vi "playback_choose_freq.vi"() -> ()   [LabVIEW 2012]
doc: "This VI will initialize the FPGA VI and read a user-defined number of samples from a DMA FIFO. When the data acquisition is complete this VI will read status information from the FPGA VI.\n\nFollow these instructions to run the VI.\n\n1. Select your RIO device from the dropdown.\n2. Set the sample period, number of samples to acquire per channel, and DMA block read size. \n\nNote: the block read size should be set to balance load on the host processor and the update rate of the user interface. A small block read size will update the user interface more often but will result in a higher load on the host processor."
uses:
  <vilib>/Analysis/3filter.llb/Butterworth Filter (DBL).vi
  <vilib>/Analysis/NI_AALBase.lvlib
panel:
  out "Selected Index":i32
  out "Ratio at Index (%)":dbl
  in  "Threshold":dbl=0.1
  out "Index 0":dbl
  out "Index 1":dbl
  out "Index 2":dbl
  out "Index 3":dbl
  in  "noise min":dbl=0.001
  out "amplitude 0":dbl
  out "amplitude 1":dbl
  out "amplitude 2":dbl
  out "amplitude 3":dbl
  in  "Portion Duration":i32=600
  in  "Altitude":dbl=2.0
  out "x":dbl
  out "y":dbl
  out "z":dbl
  out "yaw":dbl
  out "pitch":dbl
  out "Yaw Chart":dbl(graph)
  in  "Mode":T1(ring)=enum."Use Far Field"
  out "Threshold 0":dbl
  out "Threshold 1":dbl
  out "Threshold 2":dbl
  out "Threshold 3":dbl
  in  "threshold ratio":dbl=3.0
  out "bad signal?":bool
  out "ROS  Error":bool
  in  "Send to ROS":bool
  out "dt1":dbl
  out "dt2":dbl
  out "dt3":dbl
  out "Forward":dbl
  out "Sidemove":dbl
  out "Extracted signal":dbl[][](graph)
  in  "Debug":bool=TRUE
  in  "Select Frequency":dbl=24000.0
  out "frequency 2":dbl
  out "frequency 1":dbl
  out "Chosen Signal":dbl[][](graph)
  in  "Wait?":bool
  in  "Next Signal":bool
  in  "Filename":path=path "D/Recorded/US Test/Robosub day 1/pinger_in_front.tdms"
  out "Original Filtered Ch0":dbl[](graph)
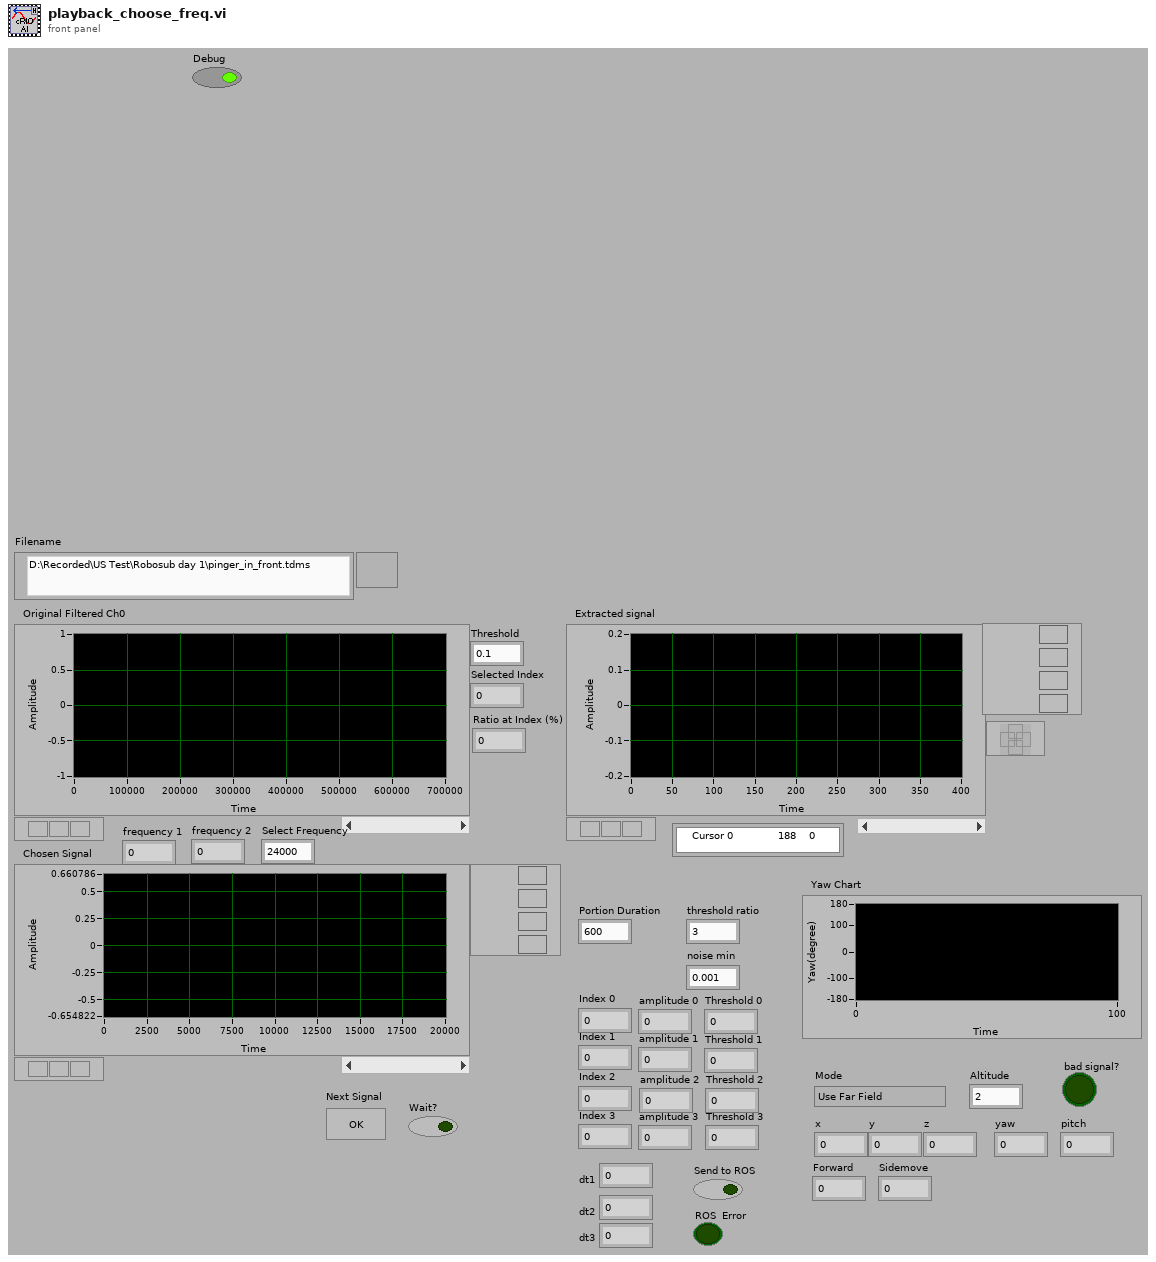
[diagram p1: front panel]
types:
  T1 = enum16{"Use Near Field", "Use Far Field", "Far Field with 3 hydrophones"}
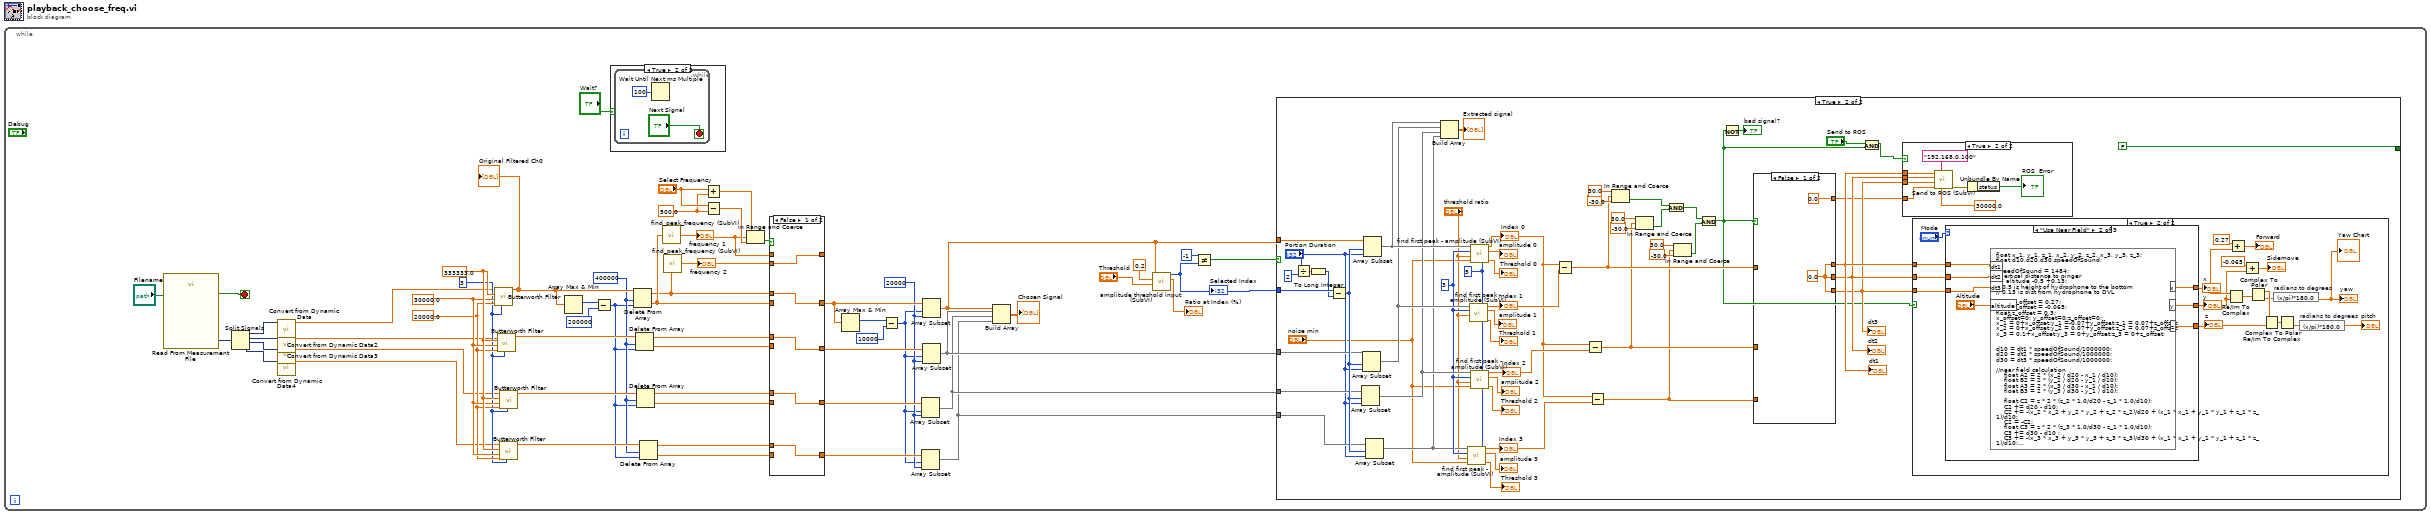
[diagram p0: block diagram]
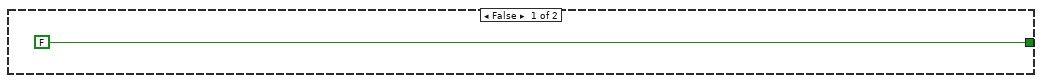
[diagram p2: hidden frame]
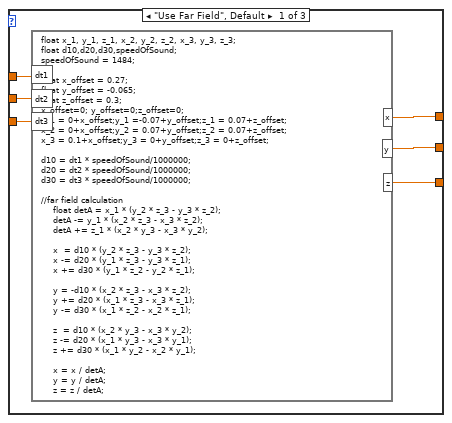
[diagram p4: hidden frame]
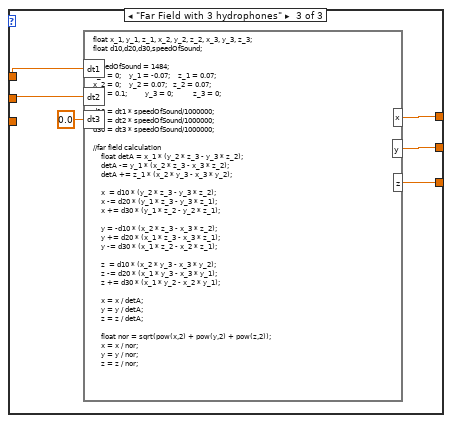
[diagram p5: hidden frame]
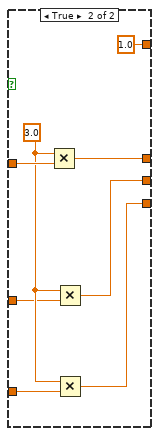
[diagram p7: hidden frame]
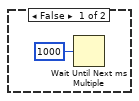
[diagram p8: hidden frame]
diagram:
  n1 = while {
    stop <- w46 stop-if-true
    w17 = 500.0
    w23 = 20000
    w37 = 400000
    w56 = 20000.0
    w57 = 30000.0
    w55 = 3
    w58 = 333333.0
    n2 = call "Read From Measurement File"("Filename"="Filename") -> ("Signals"=w50:dynamicdata, "EOF?"=w46:bool)  [unwired: 5 in, 4 out]
    n3 = Split Signals(w50) -> (w54:dynamicdata, w53:dynamicdata, w52:dynamicdata, w51:dynamicdata)  [unwired: 4 in]
    n4 = call "Convert from Dynamic Data"("Dynamic Data Type"=w54) -> ("Array"=w44:dbl[])  [unwired: 3 in]
    n5 = call "Convert from Dynamic Data2"("Dynamic Data Type"=w53) -> ("Array"=w49:dbl[])  [unwired: 3 in]
    n6 = call "Convert from Dynamic Data3"("Dynamic Data Type"=w52) -> ("Array"=w47:dbl[])  [unwired: 3 in]
    n7 = call "Convert from Dynamic Data4"("Dynamic Data Type"=w51) -> ("Array"=w48:dbl[])  [unwired: 3 in]
    n8 = call-poly <vilib>:"Butterworth Filter.vi"("order"=w55, "low cutoff freq: fl"=w56, "high cutoff freq: fh"=w57, "sampling freq: fs"=w58, "X"=w44) -> ("Filtered X"=w43:dbl[])  [unwired: 3 in, 1 out]
    "Original Filtered Ch0" <- w43
    n9 = call-poly <vilib>:"Butterworth Filter.vi"("order"=w55, "low cutoff freq: fl"=w56, "high cutoff freq: fh"=w57, "sampling freq: fs"=w58, "X"=w49) -> ("Filtered X"=w40:dbl[])  [unwired: 3 in, 1 out]
    n10 = call-poly <vilib>:"Butterworth Filter.vi"("order"=w55, "low cutoff freq: fl"=w56, "high cutoff freq: fh"=w57, "sampling freq: fs"=w58, "X"=w48) -> ("Filtered X"=w38:dbl[])  [unwired: 3 in, 1 out]
    n11 = call-poly <vilib>:"Butterworth Filter.vi"("order"=w55, "low cutoff freq: fl"=w56, "high cutoff freq: fh"=w57, "sampling freq: fs"=w58, "X"=w47) -> ("Filtered X"=w39:dbl[])  [unwired: 3 in, 1 out]
    n12 = Array Max & Min(array=w43) -> (max index (indices)=w42:i32)  [unwired: 3 out]
    n13 = Subtract(x=w42, y=200000) -> (x-y=w36:i32)
    n14 = case shown="True" "Wait?" {
      frame False {
        n15 = Wait Until Next ms Multiple(millisecond multiple=u32 1000) -> ()  [unwired: 1 out]
      }
      frame True {
        n16 = while {
          stop <- "Next Signal" stop-if-true
          n17 = Wait Until Next ms Multiple(millisecond multiple=u32 100) -> ()  [unwired: 1 out]
        }
      }
    }
    n18 = Delete From Array(array=w43, length=w37, index=w36) -> (deleted portion=w20:dbl[], array with subset deleted=w19:dbl[])
    n19 = Delete From Array(array=w40, length=w37, index=w36) -> (deleted portion=w35:dbl[], array with subset deleted=w32:dbl[])
    n20 = Delete From Array(array=w39, length=w37, index=w36) -> (deleted portion=w34:dbl[], array with subset deleted=w31:dbl[])
    n21 = Delete From Array(array=w38, length=w37, index=w36) -> (deleted portion=w33:dbl[], array with subset deleted=w30:dbl[])
    n22 = call "find_peak_frequency (SubVI).vi"("Signal"=w20) -> ("Frequency"=w13:dbl)
    "frequency 1" <- w13
    n23 = call "find_peak_frequency (SubVI).vi"("Signal"=w19) -> ("Frequency"=w12:dbl)
    "frequency 2" <- w12
    n24 = Add(x="Select Frequency", y=w17) -> (x+y=w15:dbl)
    n25 = Subtract(x="Select Frequency", y=w17) -> (x-y=w14:dbl)
    n26 = In Range and Coerce(upper limit=w15, x=w13, lower limit=w14) -> (In Range?=w16:bool)  [unwired: 1 out]
    n27 = case shown="False" w16 {
      tunnel: w20 -> [_ w180]
      tunnel: w35 -> [_ w179]
      tunnel: w34 -> [_ w178]
      tunnel: w33 -> [_ w177]
      tunnel: w19 -> [w175 _]
      tunnel: w32 -> [w174 _]
      tunnel: w31 -> [w173 _]
      tunnel: w30 -> [w172 _]
      tunnel: [w175 w180] -> w27
      tunnel: [w174 w179] -> w26
      tunnel: [w173 w178] -> w25
      tunnel: [w172 w177] -> w24
      tunnel: [w171 w176] -> _
      tunnel: w13 -> [_ w176]
      tunnel: w12 -> [w171 _]
      frame False {
      }
      frame True {
      }
    }
    n28 = Array Max & Min(array=w27) -> (max index (indices)=w28:i32)  [unwired: 3 out]
    n29 = Subtract(x=w28, y=10000) -> (x-y=w22:i32)
    n30 = Array Subset(array=w25, index=w22, length=w23) -> (w2:dbl[])
    n31 = Array Subset(array=w24, index=w22, length=w23) -> (w1:dbl[])
    n32 = Array Subset(array=w27, index=w22, length=w23) -> (w4:dbl[])
    n33 = Array Subset(array=w26, index=w22, length=w23) -> (w3:dbl[])
    n34 = Build Array(w4, w3, w2, w1) -> (→"Chosen Signal":dbl[][])
    n35 = call "amplitude threshold input (SubVI).vi"("threshold"="Threshold", "%max amplitude"=0.2, "Array"=w4) -> ("actual ratio (%)"=→"Ratio at Index (%)":dbl, "Index"=w5:i32)  [unwired: 7 in]
    "Selected Index" <- w5
    n36 = Not Equal?(x=-1, y=w5) -> (x != y?=w9:bool)
    n37 = case shown="True" w9 {
      tunnel: w3 -> [_ w111]
      tunnel: w2 -> [_ w110]
      tunnel: w1 -> [_ w109]
      tunnel: w4 -> [_ w108]
      tunnel: w5 -> [_ w107]
      tunnel: [FALSE FALSE] -> _
      frame False {
      }
      frame True {
        w61 = 5
        w73 = 3
        n38 = Divide(x="Portion Duration", y=2) -> (x/y=w104:dbl)
        n39 = To Long Integer(number=w104) -> (32bit integer=w103:i32)
        n40 = Subtract(x=w107, y=w103) -> (x-y=w112:i32)
        n41 = Array Subset(array=w110, index=w112, length="Portion Duration") -> (w74:dbl[])
        n42 = Array Subset(array=w111, index=w112, length="Portion Duration") -> (w78:dbl[])
        n43 = Array Subset(array=w108, index=w112, length="Portion Duration") -> (w80:dbl[])
        n44 = Array Subset(array=w109, index=w112, length="Portion Duration") -> (w72:dbl[])
        n45 = Build Array(w80, w78, w74, w72) -> (→"Extracted signal":dbl[][])
        n46 = call "find first peak - amplitude (SubVI).vi"("Noise length"=w61, "Noise min"="noise min", "threshold ratio"="threshold ratio", "width"=w73, "Array"=w72) -> ("Peak threshold"=→"Threshold 3":dbl, "peak amplitude"=→"amplitude 3":dbl, "Index"=w71:dbl)  [unwired: 2 in, 2 out]
        "Index 3" <- w71
        n47 = call "find first peak - amplitude (SubVI).vi"("Noise length"=w61, "threshold ratio"="threshold ratio", "width"=w73, "Array"=w78) -> ("Peak threshold"=→"Threshold 1":dbl, "peak amplitude"=→"amplitude 1":dbl, "Index"=w77:dbl)  [unwired: 3 in, 2 out]
        "Index 1" <- w77
        n48 = call "find first peak - amplitude (SubVI).vi"("Noise length"=w61, "Noise min"="noise min", "threshold ratio"="threshold ratio", "width"=w73, "Array"=w80) -> ("Peak threshold"=→"Threshold 0":dbl, "peak amplitude"=→"amplitude 0":dbl, "Index"=w67:dbl)  [unwired: 2 in, 2 out]
        "Index 0" <- w67
        n49 = call "find first peak - amplitude (SubVI).vi"("Noise length"=w61, "Noise min"="noise min", "threshold ratio"="threshold ratio", "width"=w73, "Array"=w74) -> ("Peak threshold"=→"Threshold 2":dbl, "peak amplitude"=→"amplitude 2":dbl, "Index"=w75:dbl)  [unwired: 2 in, 2 out]
        "Index 2" <- w75
        n50 = Subtract(x=w67, y=w77) -> (x-y=w99:dbl)
        n51 = Subtract(x=w67, y=w75) -> (x-y=w96:dbl)
        n52 = Subtract(x=w67, y=w71) -> (x-y=w93:dbl)
        n53 = In Range and Coerce(upper limit=30.0, x=w99, lower limit=-30.0) -> (In Range?=w92:bool)  [unwired: 1 out]
        n54 = In Range and Coerce(upper limit=30.0, x=w96, lower limit=-30.0) -> (In Range?=w91:bool)  [unwired: 1 out]
        n55 = And(x=w92, y=w91) -> (x .and. y?=w90:bool)
        n56 = In Range and Coerce(upper limit=30.0, x=w93, lower limit=-30.0) -> (In Range?=w89:bool)  [unwired: 1 out]
        n57 = And(x=w90, y=w89) -> (x .and. y?=w81:bool)
        n58 = Not(x=w81) -> (.not. x?=→"bad signal?":bool)
        n59 = case shown="False" w81 {
          tunnel: w99 -> [_ w167]
          tunnel: w96 -> [_ w165]
          tunnel: w93 -> [_ w164]
          tunnel: [w158 w163] -> w86
          tunnel: [w158 w162] -> w85
          tunnel: [w158 w161] -> w84
          tunnel: [0.0 1.0] -> w83
          frame False {
            w158 = 0.0
          }
          frame True {
            w166 = 3.0
            n60 = Multiply(x=w166, y=w167) -> (x*y=w163:dbl)
            n61 = Multiply(x=w166, y=w165) -> (x*y=w162:dbl)
            n62 = Multiply(x=w166, y=w164) -> (x*y=w161:dbl)
          }
        }
        "dt1" <- w86
        "dt2" <- w85
        "dt3" <- w84
        n63 = And(x="Send to ROS", y=w81) -> (x .and. y?=w82:bool)
        n64 = case shown="True" w82 {
          tunnel: w86 -> [_ w153]
          tunnel: w85 -> [_ w152]
          tunnel: w84 -> [_ w151]
          tunnel: w83 -> [_ w150]
          frame False {
          }
          frame True {
            n65 = call "Send to ROS (SubVI).vi"("frequency"=30000.0, "ROS IP"="192.168.0.100", "Good signal?"=w150, "dt 3"=w151, "dt2"=w152, "dt 1"=w153) -> ("error out"=w156:errorcluster)  [unwired: 5 in]
            n66 = Unbundle By Name(w156) -> ("status"=→"ROS  Error":bool)
          }
        }
        n67 = case shown="True" w81 {
          tunnel: w86 -> [_ w121]
          tunnel: w85 -> [_ w120]
          tunnel: w84 -> [_ w119]
          frame False {
          }
          frame True {
            n68 = case shown="\"Use Near Field\"" "Mode" {
              tunnel: [w136 w143 w148] -> w118
              tunnel: [w135 w142 w147] -> w115
              tunnel: [w134 w141 w146] -> w125
              tunnel: w121 -> [w133 w139 w145]
              tunnel: w120 -> [w132 w138 w144]
              tunnel: w119 -> [w131 w137 _]
              frame "Use Far Field", Default {
                n69 = formula code="float x_1, y_1, z_1, x_2, y_2, z_2, x_3, y_3, z_3;\nfloat d10,d20,d30,speedOfSound;\nspeedOfSound = 1484;\n\nfloat x_offset = 0.27;\nfloat y_offset = -0.065;\nfloat z_offset = 0.3;\nx_offset=0; y_offset=0;z_offset=0;\nx_1 = 0+x_offset;y_1 =-0.07+y_offset;z_1 = 0.07+z_offset;\nx_2 = 0+x_offset;y_2 = 0.07+y_offset;z_2 = 0.07+z_offset;\nx_3 = 0.1+x_offset;y_3 = 0+y_offset;z_3 = 0+z_offset;\n\nd10 = dt1 * speedOfSound/1000000;\nd20 = dt2 * speedOfSound/1000000;\nd30 = dt3 * speedOfSound/1000000;\n\n//far field calculation\n    float detA = x_1 * (y_2 * z_3 - y_3 * z_2);\n    detA -= y_1 * (x_2 * z_3 - x_3 * z_2);\n    detA += z_1 * (x_2 * y_3 - x_3 * y_2);\n\n    x  = d10 * (y_2 * z_3 - y_3 * z_2);\n    x -= d20 * (y_1 * z_3 - y_3 * z_1);\n    x += d30 * (y_1 * z_2 - y_2 * z_1);\n\n    y = -d10 * (x_2 * z_3 - x_3 * z_2);\n    y += d20 * (x_1 * z_3 - x_3 * z_1);\n    y -= d30 * (x_1 * z_2 - x_2 * z_1);\n\n    z  = d10 * (x_2 * y_3 - x_3 * y_2);\n    z -= d20 * (x_1 * y_3 - x_3 * y_1);\n    z += d30 * (x_1 * y_2 - x_2 * y_1);\n\n    x = x / detA;\n    y = y / detA;\n    z = z / detA;\n\n    float nor = sqrt(pow(x,2) + pow(y,2) + pow(z,2));\n    x = x / nor;\n    y = y / nor;\n    z = z / nor;"("dt1"=w133, "dt2"=w132, "dt3"=w131) -> ("x"=w136:dbl, "y"=w135:dbl, "z"=w134:dbl)
              }
              frame "Use Near Field" {
                n70 = formula code="float x_1, y_1, z_1, x_2, y_2, z_2, x_3, y_3, z_3;\nfloat d10,d20,d30,speedOfSound;\n\nspeedOfSound = 1484;\n//vertical distance to pinger\nz= altitude -0.5 +0.13;\n// 0.5 is height of hydrophone to the bottom\n// 0.13 is dist from hydrophone to DVL\n\nfloat x_offset = 0.27;\nfloat y_offset = -0.065;\nfloat z_offset = 0.3;\nx_offset=0; y_offset=0;z_offset=0;\nx_1 = 0+x_offset;y_1 =-0.07+y_offset;z_1 = 0.07+z_offset;\nx_2 = 0+x_offset;y_2 = 0.07+y_offset;z_2 = 0.07+z_offset;\nx_3 = 0.1+x_offset;y_3 = 0+y_offset;z_3 = 0+z_offset;\n\n\nd10 = dt1 * speedOfSound/1000000;\nd20 = dt2 * speedOfSound/1000000;\nd30 = dt3 * speedOfSound/1000000;\n\n//near field calculation\n    float A2 = 2 * (x_2 / d20 - x_1 / d10);\n    float B2 = 2 * (y_2 / d20 - y_1 / d10);\n    float A3 = 2 * (x_3 / d30 - x_1 / d10);\n    float B3 = 2 * (y_3 / d30 - y_1 / d10);\n    \n    float C2 = z * 2 * (z_2 * 1.0/d20 - z_1 * 1.0/d10);\n    C2 += d20 - d10;\n    C2 += -(x_2 * x_2 + y_2 * y_2 + z_2 * z_2)/d20 + (x_1 * x_1 + y_1 * y_1 + z_1 * z_1)/d10;\n    C2 = -C2;\n    float C3 = z * 2 * (z_3 * 1.0/d30 - z_1 * 1.0/d10);\n    C3 += d30 - d10 ;\n    C3 += -(x_3 * x_3 + y_3 * y_3 + z_3 * z_3)/d30 + (x_1 * x_1 + y_1 * y_1 + z_1 * z_1)/d10;\n    C3 = -C3;\n\n    if (A2*B3 == A3*B2) {\n        x = 0;\n        y = 0;\n    }\n    else {\n        x = (C2 * B3 - C3 * B2) / (A2 * B3 - A3 * B2);\n        y = (C3 * A2 - C2 * A3) / (B3 * A2 - B2 * A3);\n    }"("dt1"=w139, "dt2"=w138, "dt3"=w137, "altitude"="Altitude") -> ("x"=w143:dbl, "y"=w142:dbl, "z"=w141:dbl)
              }
              frame "Far Field with 3 hydrophones" {
                n71 = formula code="float x_1, y_1, z_1, x_2, y_2, z_2, x_3, y_3, z_3;\nfloat d10,d20,d30,speedOfSound;\n\nspeedOfSound = 1484;\nx_1 = 0;    y_1 = -0.07;    z_1 = 0.07;\nx_2 = 0;    y_2 = 0.07;   z_2 = 0.07;\nx_3 = 0.1;         y_3 = 0;          z_3 = 0;\n\nd10 = dt1 * speedOfSound/1000000;\nd20 = dt2 * speedOfSound/1000000;\nd30 = dt3 * speedOfSound/1000000;\n\n//far field calculation\n    float detA = x_1 * (y_2 * z_3 - y_3 * z_2);\n    detA -= y_1 * (x_2 * z_3 - x_3 * z_2);\n    detA += z_1 * (x_2 * y_3 - x_3 * y_2);\n\n    x  = d10 * (y_2 * z_3 - y_3 * z_2);\n    x -= d20 * (y_1 * z_3 - y_3 * z_1);\n    x += d30 * (y_1 * z_2 - y_2 * z_1);\n\n    y = -d10 * (x_2 * z_3 - x_3 * z_2);\n    y += d20 * (x_1 * z_3 - x_3 * z_1);\n    y -= d30 * (x_1 * z_2 - x_2 * z_1);\n\n    z  = d10 * (x_2 * y_3 - x_3 * y_2);\n    z -= d20 * (x_1 * y_3 - x_3 * y_1);\n    z += d30 * (x_1 * y_2 - x_2 * y_1);\n\n    x = x / detA;\n    y = y / detA;\n    z = z / detA;\n\n    float nor = sqrt(pow(x,2) + pow(y,2) + pow(z,2));\n    x = x / nor;\n    y = y / nor;\n    z = z / nor;"("dt1"=w145, "dt2"=w144, "dt3"=0.0) -> ("x"=w148:dbl, "y"=w147:dbl, "z"=w146:dbl)
              }
            }
            "x" <- w118
            "y" <- w115
            "z" <- w125
            n72 = Re/Im To Complex(1:w115, 2:w118) -> (0:w123:cdb)
            n73 = Add(x=0.27, y=w118) -> (x+y=→"Forward":dbl)
            n74 = Add(x=-0.065, y=w115) -> (x+y=→"Sidemove":dbl)
            n75 = Complex To Polar(r * e^(i*theta)=w123) -> (r=w126:dbl, theta=w124:dbl)
            n76 = Re/Im To Complex(1:w125, 2:w126) -> (0:w127:cdb)
            n77 = expression code="(x/pi)*180.0"(w124) -> (→"yaw" →"Yaw Chart":dbl)
            n78 = Complex To Polar(r * e^(i*theta)=w127) -> (theta=w129:dbl)  [unwired: 1 out]
            n79 = expression code="(x/pi)*180.0"(w129) -> (→"pitch":dbl)
          }
        }
      }
    }
  }
